vi "parseRS232.vi"(8 "error in (no error)":errorcluster, 11 "Model in":refnum<class "Model.lvclass">) -> (0 "error out":errorcluster, 3 "Model out":refnum<class "Model.lvclass">)   [LabVIEW 2016, in "Model.lvclass"]
uses:
  Model.lvclass
  Model.lvclass/Model.ctl
  Resources/FPGA/FPGA.lvclass
  Common_RT_T7Inclinometer/T7Inclinometer/T7Inclinometer.lvclass
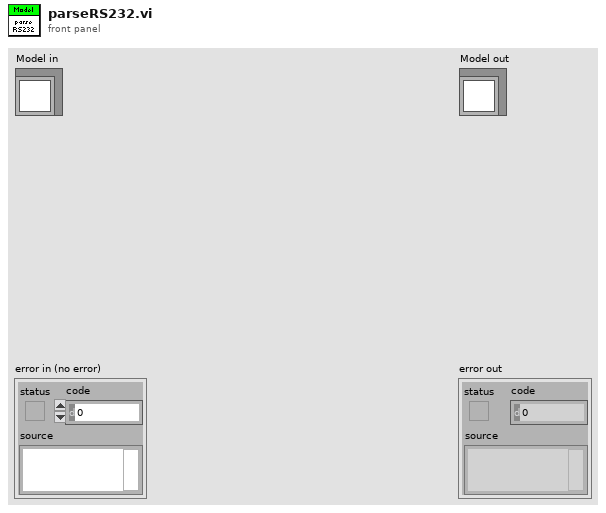
[diagram p1: front panel]
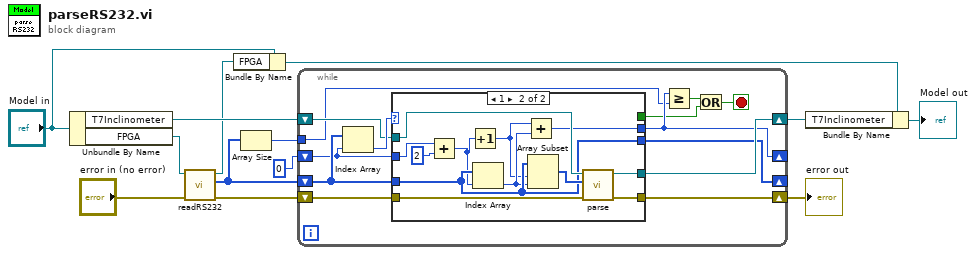
[diagram p0: block diagram]
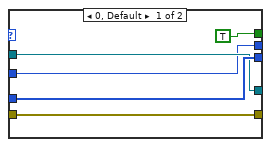
[diagram p2: hidden frame]
diagram:
  n1 = Unbundle By Name("Model in") -> ("T7Inclinometer"=w11:refnum<class "T7Inclinometer.lvclass">, "FPGA"=w13:refnum<class "FPGA.lvclass">)
  n2 = call "readRS232.vi"("error in (no error)"="error in (no error)", "FPGA in"=w13) -> ("error out"=w9:errorcluster, "Data"=w2:u8[], "FPGA out"=w6:refnum<class "FPGA.lvclass">)  [unwired: 7 in]
  n3 = Bundle By Name(cluster="Model in", "FPGA"=w6) -> (w5:refnum<class "Model.lvclass">)
  n4 = Array Size(array=w2) -> (size(s)=w1:i32)
  n5 = while {
    shift-right: [w18] -> _
    shift-left: 0 -> [w24]
    shift-right: [w19] -> _
    shift-left: w2 -> [w25]
    shift-right: [w22] -> w4
    shift-left: w11 -> [w23]
    shift-right: [w20] -> w8
    shift-left: w9 -> [w21]
    tunnel: w1 -> [w17]
    stop <- w14 stop-if-true
    n6 = Index Array(array=w25, index=w24) -> (element=w26:u8)
    n7 = case shown="1" w26 {
      tunnel: w25 -> [w31 w36]
      tunnel: w24 -> [w27 w43]
      tunnel: w23 -> [w30 w41]
      tunnel: [w30 w39] -> w22
      tunnel: w21 -> [w29 w38]
      tunnel: [w29 w37] -> w20
      tunnel: [w31 w36] -> w19
      tunnel: [w27 w34] -> w18
      tunnel: [TRUE _] -> w15
      frame 0, Default {
      }
      frame 1 {
        n8 = Add(x=w43, y=2) -> (x+y=w33:i32)
        n9 = Increment(x=w33) -> (x+1=w32:i32)
        n10 = Index Array(array=w36, index=w33) -> (element=w35:u8)
        n11 = Add(x=w32, y=w35) -> (x+y=w34:i32)
        n12 = Array Subset(array=w36, index=w32, length=w35) -> (w40:u8[])
        n13 = call "parse.vi"("error in (no error)"=w38, "Message"=w40, "T7Inclinometer in"=w41) -> ("error out"=w37:errorcluster, "T7Inclinometer out"=w39:refnum<class "T7Inclinometer.lvclass">)  [unwired: 6 in, 1 out]
      }
    }
    n14 = Greater Or Equal?(x=w18, y=w17) -> (x >= y?=w16:bool)
    n15 = Or(x=w16, y=w15) -> (x .or. y?=w14:bool)
  }
  "error out" <- w8
  n16 = Bundle By Name(cluster=w5, "T7Inclinometer"=w4) -> (→"Model out":refnum<class "Model.lvclass">)
